vi "asdsad.vi"() -> ()   [LabVIEW 2018]
uses:
  trlamp.ctl
panel:
  in  "열거형":T1
  out "Red":bool
  out "Orange":bool
  out "Green":bool
  in  "Exit Button":bool
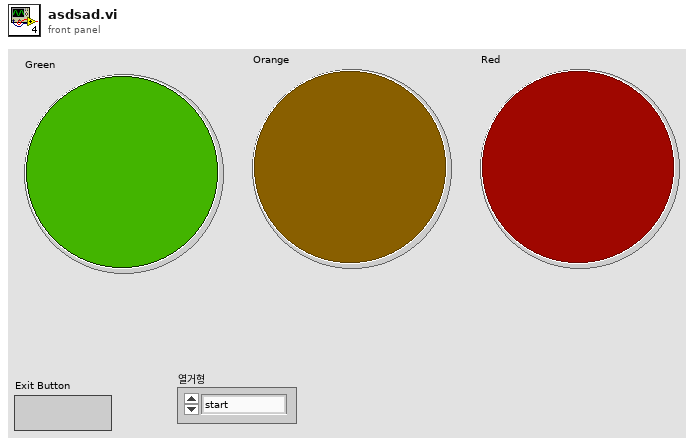
[diagram p1: front panel]
types:
  T1 = typedef "trlamp.ctl" = enum16{"start", "init", "green", "orange", "red", "idle", "stop"}
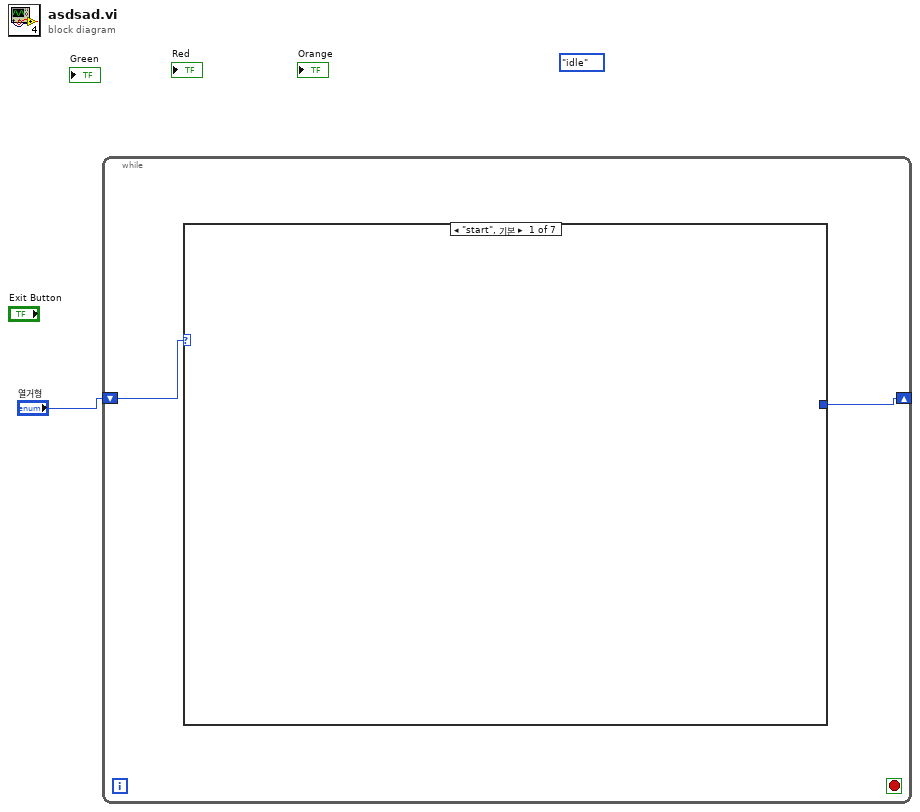
[diagram p0: block diagram]
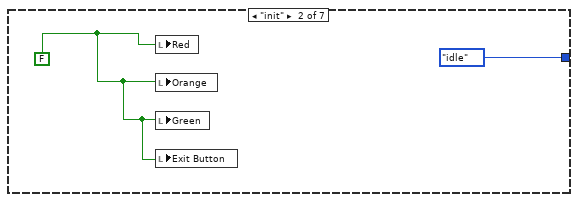
[diagram p2: hidden frame]
diagram:
  (unwired) trlamp."idle" ("열거형 2")
  n1 = while {
    shift-right: [w2] -> _
    shift-left: "열거형" -> [w3]
    stop <- _ stop-if-true
    n2 = case shown="\"start\", 기본" w3 {
      tunnel: [_ trlamp."idle" ("열거형 2") _ _ _ _ _] -> w2
      frame "start", Default {
      }
      frame "init" {
        w5 = FALSE
        n3 = local write "Red"(w5) -> ()
        n4 = local write "Orange"(w5) -> ()
        n5 = local write "Green"(w5) -> ()
        n6 = local write "Exit Button"(w5) -> ()
      }
      frame "green" {
      }
      frame "orange" {
      }
      frame "red" {
      }
      frame "idle" {
      }
      frame "stop" {
      }
    }
  }
